vi "Localized Strings.vi"() -> ()   [LabVIEW 2020, in "AF Debug.lvlib"]
uses:
  AF Debug.lvlib
panel:
  in  "Custom Trace Format String":string="AF:  %1$s%2$s %3$s"
  in  "Stopped Time-Delayed Message Format String":string="AF:  %1$s %2$s %3$s"
  in  "has stopped":string="has stopped"
  in  "Stopped Actor Format String":string="AF:  %1$s %2$s %3$s"
  in  "skipped a message":string="skipped a message"
  in  "Time-Delayed Message Skipped Format String":string="AF:  %1$s %2$s %3$s"
  in  "received":string="received"
  in  "Received Message Format String":string="AF:  %1$s %2$s %3$s %4$s"
  in  "for":string="for"
  in  "created Time-Delayed Message":string="created Time-Delayed Message"
  in  "New Time-Delayed Message Format String":string="AF:  %1$s%2$s %3$s %4$s %5$s %6$s"
  in  "of type":string="of type"
  in  "created Actor":string="created Actor"
  in  "New Actor Format String":string="AF:  %1$s%2$s %3$s %4$s %5$s %6$s"
  in  "to":string="to"
  in  "sent":string="sent"
  in  "Message Format String":string="AF:  %1$s%2$s %3$s %4$s %5$s %6$s %7$s"
  in  "Time-Delayed Message":string="Time-Delayed Message"
  in  "Non-actor":string="Unregistered Entity"
  in  "Actor":string="Actor"
  in  "dropped":string="dropped"
  in  "Dropped Message Format String":string="AF:  %1$s%2$s %3$s %4$s"
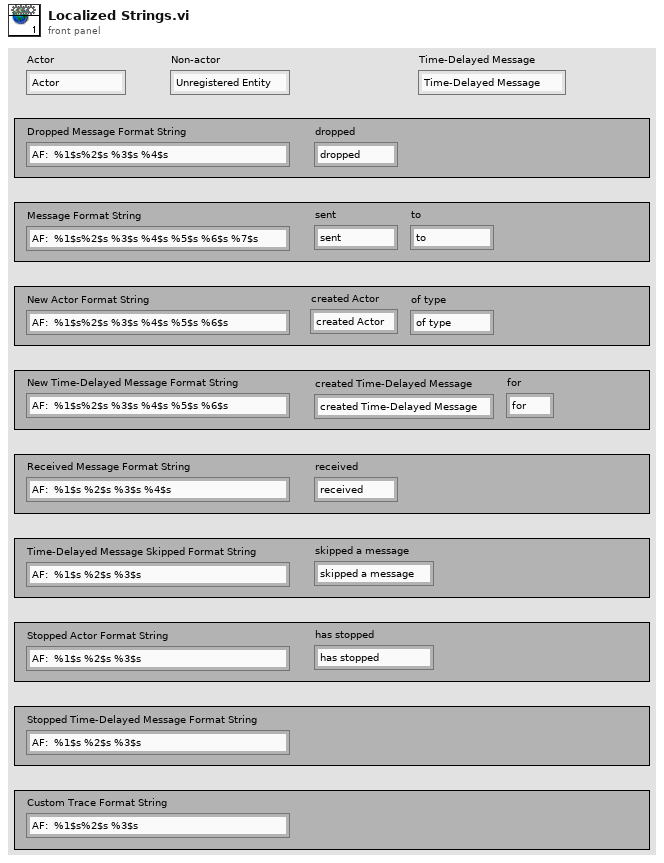
[diagram p1: front panel]
diagram:
